vi "SetGateHeight.vi"(8 "错误输入（无错误）":errorcluster, 10 "滤波模式索引值":u16, 11 "SelGateType":i32) -> (0 "错误输出":errorcluster)   [LabVIEW 2014]
uses:
  ZXUTConfigMgr.dll
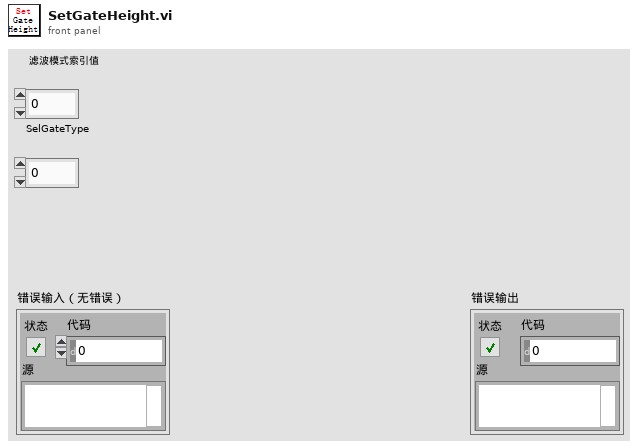
[diagram p1: front panel]
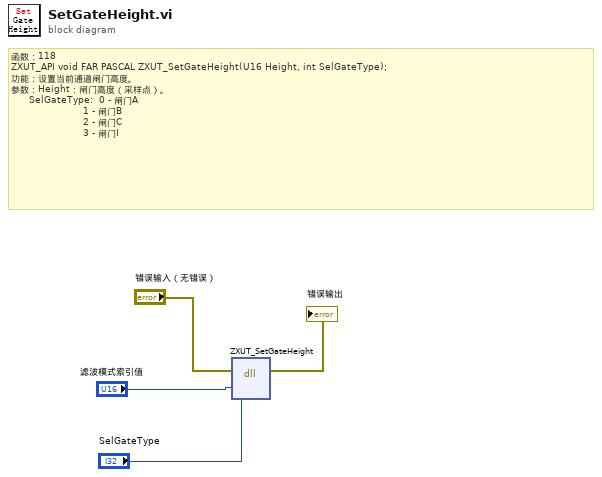
[diagram p0: block diagram]
diagram:
  # "函数：118\nZXUT_API void\tFAR PASCAL ZXUT_SetGateHeight(U16 Height, int SelGateType);\n功能：设置当前通道闸门高度。\n参数：Height：闸门高度（采样点）。\n      SelGateType:  0 - 闸门A \n                        1 - 闸门B\n                        2 - 闸门C\n                        3 - 闸门I"
  n1 = dll-call lib="PTH2eabs D软件超声实时监测软件ZXUTAppDemo(华南理工V02.00)X86DllZXUTConfigMgr.dll" fn="ZXUT_SetGateHeight"(error in="错误输入（无错误）", "Height"="滤波模式索引值", "SelGateType"="SelGateType") -> (error out=→"错误输出":errorcluster)  [unwired: 5 in, 1 out]
